vi "SetProcessFullName.vi"(8 "error in":errorcluster, 10 "ProcessFullName":string, 11 "ProcessRun in":refnum<class "ProcessRun.lvclass">) -> (0 "error out":errorcluster, 3 "ProcessRun out":refnum<class "ProcessRun.lvclass">)   [LabVIEW 2021, in "ProligentXMLGenerator.lvlib" / "ProcessRun.lvclass"]
doc: "Defines the name of the process for this process run.\n\n\"[Root Process/][[Path/]...]Name\"\nEach path strings and the name are limited to 64 characters and the total string provided is limited to 1900 characters\n\nWARNING:\n\nSince the '/' character is the hierarchy delimiter, if a path string contains a '/' character it will be interpreted as\na new hierarchy. It is therefore suggested to replace '/' by '-' in all your path components to keep the expected hierarchy.\nFor example, if you have a sequence named 'PASS/FAIL' and you don't substitude '/' by '-', the 'PASS' would be interpreted\nas a sequence category while 'FAIL' would be the name of a sequence. If you do the suggested substitution, the name of\nthe sequence would be interpreted as 'PASS-FAIL' without any category."
uses:
  ProcessRun.lvclass
  ProcessRun.lvclass/ProcessRun.ctl
  Base/ProcessFullName/ProcessFullName.lvclass
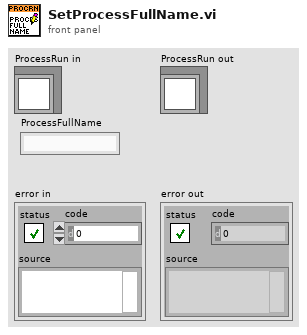
[diagram p1: front panel]
types:
  T1 = typedef "ProligentXMLGenerator.lvlib/ProcessRun.lvclass/Data.ctl" = cluster{"Name":string, "OperationRuns":refnum<class "OperationRun.lvclass">[], "OperationCycles":refnum<class "OperationCycle.lvclass">[], "FailureReferences":refnum<class "FailureReference.lvclass">[], "CustomData":refnum<class "CustomData.lvclass">, "ProcessRunId":refnum<class "Guid.lvclass">, "ProcessFullName":refnum<class "ProcessFullName.lvclass">, "ProcessVersion":refnum<class "NonEmptyString_64.lvclass">, "ProductUnitIdentifier":refnum<class "NonEmptyString_50.lvclass">, "ProductFullName":refnum<class "FullName.lvclass">, "ProcessRunStatus":refnum<class "ExecutionStatus.lvclass">, "ProcessRunStartTime":refnum<class "DateTime.lvclass">, "ProcessRunEndTime":refnum<class "DateTime.lvclass">, "ProcessMode":refnum<class "NonEmptyString_64.lvclass">, "TimeZoneInfoId":string}
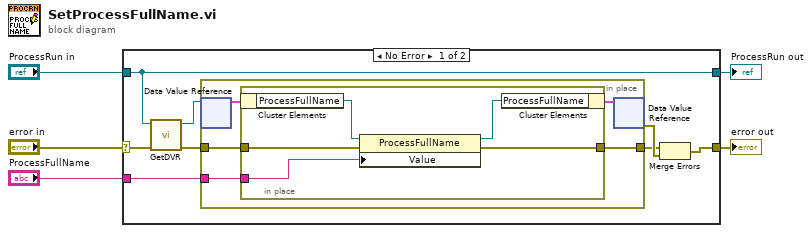
[diagram p0: block diagram]
diagram:
  n1 = case shown="No Error" "error in" {
    selector: "error in" -> [w11 w24]
    tunnel: "ProcessRun in" -> [w6 w25]
    tunnel: [w8 w24] -> w3
    tunnel: "ProcessFullName" -> [w7 _]
    tunnel: [w6 w25] -> w1
    frame No Error {
      n2 = call "GetDVR.vi"("error in"=w11, "ProcessRun"=w6) -> ("error out"=w10:errorcluster, "DVRReference"=w12:refnum<data-value>)  [unwired: 8 in]
      n3 = in-place "In Place Element Structure" {
        in-place-border: w10 -> [w18]
        in-place-border: [w17] -> w9
        in-place-border: w7 -> [w16]
        n4 = in-place-dvr #1(w12) -> (w15:T1)  [unwired: 1 out]
        n5 = in-place "In Place Element Structure" {
          in-place-border: w18 -> [w23]
          in-place-border: [w22] -> w17
          in-place-border: w16 -> [w21]
          n6 = in-place-cluster #2(w15) -> ("ProcessFullName"=w19:refnum<class "ProcessFullName.lvclass">)
          n7 = property on="Property Node" class="ProcessFullName"(reference=w19, error in=w23, "Value"=w21) -> (reference out=w20:refnum<class "ProcessFullName.lvclass">, error out=w22:errorcluster)
          n8 = in-place-cluster #2("ProcessFullName"=w20) -> (w14:T1)
        }
        n9 = in-place-dvr #1(w14) -> (w13:errorcluster)  [unwired: 1 out]
      }
      n10 = Merge Errors(w9, w13) -> (w8:errorcluster)
    }
    frame Error {
    }
  }
  "error out" <- w3
  "ProcessRun out" <- w1
